vi "VI Scripting Create Path.vi"(5 "Porition":cluster{dbl[], dbl[]}[](array[cluster]), 7 "Name":string, 8 "path":T2[](array[typedef]), 9 "right":T1[](array[typedef]), 10 "left":T1[](array[typedef]), 11 "VI in":refnum<vi>) -> ()   [LabVIEW 2016]
uses:
  VIs/Waypoint.ctl
  VIs/Segment.ctl
  <vilib>/LabVIEW Icon API/API_Rectangle Dimension.ctl
  <vilib>/LabVIEW Icon API/API_Text.ctl
  <vilib>/LabVIEW Icon API/LabVIEW Icon API.lvlib
  Pathfinder.lvlib
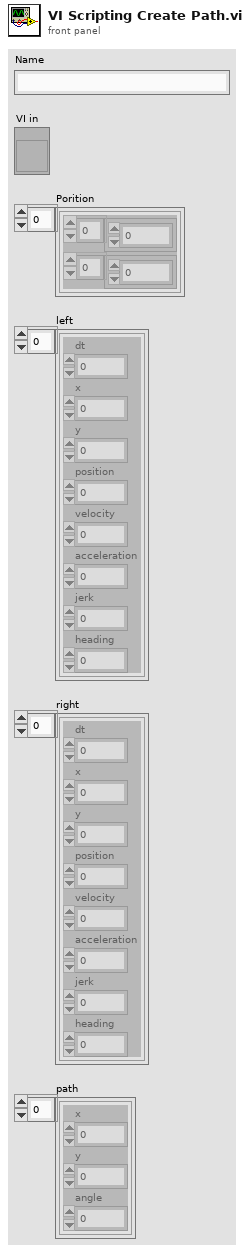
[diagram p1: front panel]
types:
  T1 = typedef "Pathfinder.lvlib/Segment.ctl" = cluster{"dt":dbl, "x":dbl, "y":dbl, "position":dbl, "velocity":dbl, "acceleration":dbl, "jerk":dbl, "heading":dbl}
  T2 = typedef "Pathfinder.lvlib/Waypoint.ctl" = cluster{"x":dbl, "y":dbl, "angle":dbl}
  T3 = typedef "LabVIEW Icon API.lvlib/API_Text.ctl" = cluster{"Line 1 text":string, "Line 2 text":string, "Line 3 text":string, "Line 4 text":string}
  T4 = typedef "LabVIEW Icon API.lvlib/API_Rectangle Dimension.ctl" = cluster{"Width":i16, "Height":i16}
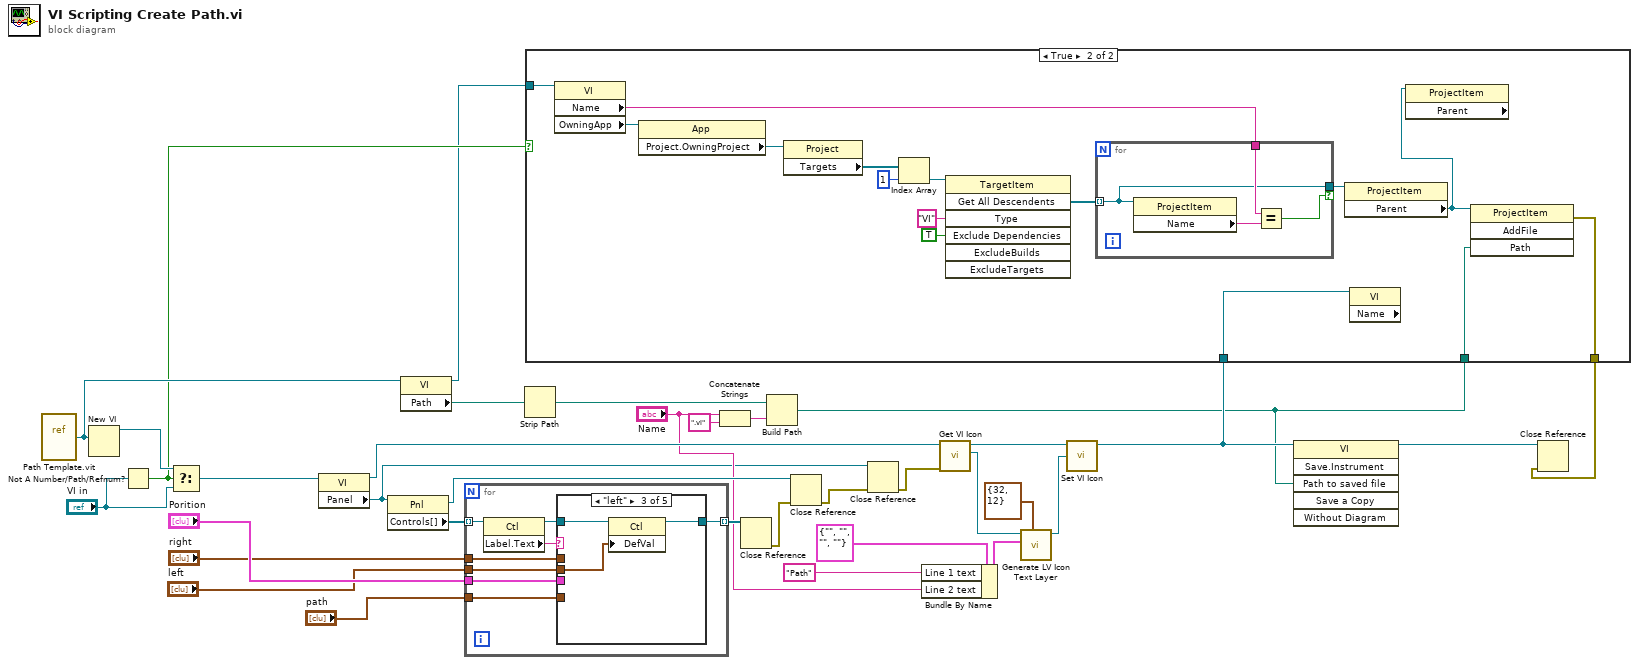
[diagram p0: block diagram]
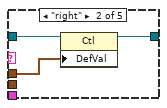
[diagram p4: hidden frame]
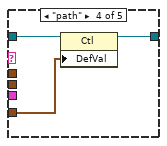
[diagram p5: hidden frame]
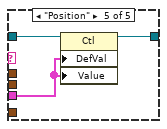
[diagram p6: hidden frame]
diagram:
  n1 = vi-ref "Path Template.vit"() -> (w7:refnum<vi>)
  n2 = New VI(10:w7) -> (3:w9:refnum<vi>)  [unwired: 6 in, 1 out]
  n3 = Not A Number/Path/Refnum?(number/path/refnum="VI in") -> (NaN/Path/Refnum?=w6:bool)
  n4 = Select(t=w9, s=w6, f="VI in") -> (s? t:f=w8:refnum<vi>)
  n5 = property class="VI"(reference=w8) -> (reference out=w34:refnum<vi>, "Panel"=w12:refnum<vi>)  [unwired: 1 in, 1 out]
  n6 = property class="Pnl"(reference=w12) -> (reference out=w21:refnum<vi>, "Controls[]"=w15:refnum<vi>[])  [unwired: 1 in, 1 out]
  n7 = property class="VI"(reference=w7) -> (reference out=w5:refnum<vi>, "Path"=w22:path)  [unwired: 1 in, 1 out]
  n8 = for {
    tunnel: w15 -> [w42] mode=indexing
    tunnel: "right" -> [w39]
    tunnel: "left" -> [w38]
    tunnel: "Porition" -> [w37]
    tunnel: [w36] -> w19 mode=indexing
    tunnel: "path" -> [w35]
    n9 = property class="Ctl"(reference=w42) -> (reference out=w40:refnum<vi>, "Label.Text"=w41:string)  [unwired: 1 in, 1 out]
    n10 = case shown="\"left\"" w41 {
      tunnel: w40 -> [w43 w46 w49 w52 w55]
      tunnel: w39 -> [_ w45 _ _ _]
      tunnel: w38 -> [_ _ w48 _ _]
      tunnel: w37 -> [_ _ _ _ w53]
      tunnel: [w43 w44 w47 w51 w54] -> w36
      tunnel: w35 -> [_ _ _ w50 _]
      frame Default {
      }
      frame "right" {
        n11 = property class="Ctl"(reference=w46, "DefVal"=w45) -> (reference out=w44:refnum<vi>)  [unwired: 1 in, 1 out]
      }
      frame "left" {
        n12 = property class="Ctl"(reference=w49, "DefVal"=w48) -> (reference out=w47:refnum<vi>)  [unwired: 1 in, 1 out]
      }
      frame "path" {
        n13 = property class="Ctl"(reference=w52, "DefVal"=w50) -> (reference out=w51:refnum<vi>)  [unwired: 1 in, 1 out]
      }
      frame "Position" {
        n14 = property class="Ctl"(reference=w55, "DefVal"=w53, "Value"=w53) -> (reference out=w54:refnum<vi>)  [unwired: 1 in, 1 out]
      }
    }
  }
  n15 = Strip Path(path=w22) -> (stripped path=w25:path)  [unwired: 1 out]
  n16 = Concatenate Strings("Name", ".vi" ("string")) -> (w23:string)
  n17 = Close Reference(reference=w19) -> (error out=w20:errorcluster)  [unwired: 1 in]
  n18 = Build Path(base path=w25, name or relative path=w23) -> (appended path=w1:path)
  n19 = Close Reference(reference=w21, error in (no error)=w20) -> (error out=w13:errorcluster)
  n20 = Close Reference(reference=w12, error in (no error)=w13) -> (error out=w11:errorcluster)
  n21 = Bundle By Name(cluster=T3 {"Line 1 text"="", "Line 2 text"="", "Line 3 text"="", "Line 4 text"=""} ("Text"), "Line 1 text"="Path", "Line 2 text"="Name") -> (w32:T3)
  n22 = call <vilib>:"Get VI Icon.vi"("error in (no error)"=w11, "VI Refnum in"=w34) -> ("Icon"=w28:refnum<class "Icon.lvclass">, "VI Refnum out"=w27:refnum<vi>)  [unwired: 7 in, 1 out]
  n23 = call <vilib>:"Generate LV Icon Text Layer.vi"("Rectangle dimension (32,32)"=T4 {"Width"=32, "Height"=12}, "Text"=w32, "Icon in"=w28) -> ("Icon out"=w29:refnum<class "Icon.lvclass">)  [unwired: 7 in, 1 out]
  n24 = call <vilib>:"Set VI Icon.vi"("Icon"=w29, "VI Refnum in"=w27) -> ("VI Refnum out"=w2:refnum<vi>)  [unwired: 8 in, 1 out]
  n25 = case shown="True" w6 {
    tunnel: w5 -> [_ w69]
    tunnel: [_ w59] -> w3
    tunnel: w2 -> [_ w58]
    tunnel: w1 -> [_ w56]
    frame False {
    }
    frame True {
      n26 = property class="VI"(reference=w69) -> ("Name"=w61:string, "OwningApp"=w68:refnum<vi>)  [unwired: 1 in, 2 out]
      n27 = property class="App"(reference=w68) -> ("Project.OwningProject"=w70:refnum<vi>)  [unwired: 1 in, 2 out]
      n28 = property class="Project"(reference=w70) -> ("Targets"=w67:refnum<vi>[])  [unwired: 1 in, 2 out]
      n29 = Index Array(array=w67, index=1) -> (element=w65:refnum<vi>)
      n30 = invoke class="TargetItem" method="Get All Descendents"(reference=w65, "Type"="VI", "Exclude Dependencies"=TRUE ("ExcludeDependencies")) -> ("All Descendents"=w62:refnum<vi>[])  [unwired: 4 in, 6 out]
      n31 = for {
        tunnel: w62 -> [w72] mode=indexing
        tunnel: w61 -> [w73]
        tunnel: [w72] -> w60 if=w71
        n32 = property class="ProjectItem"(reference=w72) -> ("Name"=w74:string)  [unwired: 1 in, 2 out]
        n33 = Equal?(x=w73, y=w74) -> (x = y?=w71:bool)
      }
      n34 = property class="ProjectItem"(reference=w60) -> ("Parent"=w57:refnum<vi>)  [unwired: 1 in, 2 out]
      n35 = property class="VI" props=["Name"](reference=w58) -> ()  [unwired: 1 in, 3 out]
      n36 = property class="ProjectItem" props=["Parent"](reference=w57) -> ()  [unwired: 1 in, 3 out]
      n37 = invoke class="ProjectItem" method="AddFile"(reference=w57, "Path"=w56) -> (error out=w59:errorcluster)  [unwired: 2 in, 3 out]
    }
  }
  n38 = invoke class="VI" method="Save.Instrument"(reference=w2, "Path to saved file"=w1) -> (reference out=w4:refnum<vi>)  [unwired: 4 in, 5 out]
  n39 = Close Reference(reference=w4, error in (no error)=w3) -> ()  [unwired: 1 out]
